vi "Flatten to String.vi"(8 "error in (no error)":errorcluster, 9 "priority":i32, 10 "Message":refnum<class "Message.lvclass">, 11 "Flattener in":refnum<class "Serializable Flattener.lvclass">) -> (0 "error out":errorcluster, 2 "Flattened String":string, 3 "Flattener out":refnum<class "Serializable Flattener.lvclass">)   [LabVIEW 2020, in "Serializer.lvlib" / "Serializable Flattener.lvclass"]
uses:
  Serializable Flattener.lvclass
  <vilib>/ActorFramework/Message/Message.lvclass
  Serializable Message/Serializable Msg.lvclass
  Cache Manager/Cache Manager.lvclass/Cache Manager.ctl
  Serializable Message/Serializable Msg.lvclass/Serializable Msg.ctl
  Serializable Message/Make Header Array.vi
  <vilib>/Utility/LVClass/Get LV Class Name.vi
  Serializable Flattener.lvclass/Serializable Flattener.ctl
  Cache Manager/Cache Manager.lvclass
panel:
  out "Elapsed time":u32
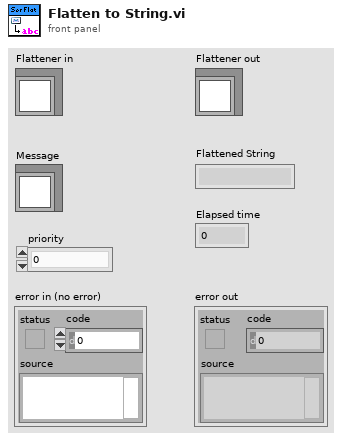
[diagram p1: front panel]
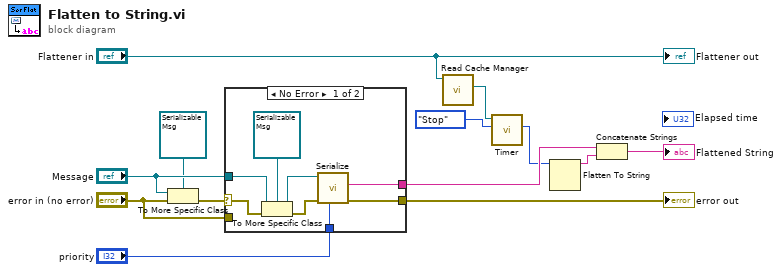
[diagram p0: block diagram]
diagram:
  n1 = To More Specific Class(target class=refnum<class "Serializable Msg.lvclass"> refnum ("Serializable Message in"), reference="Message", error in="error in (no error)") -> (error out=w9:errorcluster)  [unwired: 1 out]
  n2 = case shown="No Error" w9 {
    selector: w9 -> [w17 _]
    tunnel: [w19 w22] -> w13
    tunnel: [w18 _] -> w5
    tunnel: "Message" -> [w15 _]
    tunnel: "priority" -> [w14 _]
    tunnel: "error in (no error)" -> [_ w22]
    frame No Error {
      n3 = To More Specific Class(target class=refnum<class "Serializable Msg.lvclass"> refnum ("Serializable Message in"), reference=w15, error in=w17) -> (specific class reference=w16:refnum<class "Serializable Msg.lvclass">, error out=w21:errorcluster)
      n4 = call "Serialize.vi"("priority"=w14, "error in (no error)"=w21, "Serializable Message in"=w16) -> ("error out"=w19:errorcluster, "Serialized Message"=w18:string)  [unwired: 7 in]
    }
    frame Error {
    }
  }
  "error out" <- w13
  n5 = call-dynamic "Read Cache Manager.vi"("Message Flattener in"="Flattener in") -> ("Cache Manager DVR.lvclass"=w3:refnum<class "Cache Manager.lvclass">)  [unwired: 9 in, 1 out]
  n6 = call "Timer.vi"("Action"=enum16{"Stop", "Start", ""}."Stop", "Cache Manager DVR in"=w3) -> ("Elapsed time (ms)"=w1:u32)  [unwired: 7 in, 2 out]
  n7 = Flatten To String(anything=w1) -> (data string=w4:string)  [unwired: 3 in, 2 out]
  n8 = Concatenate Strings(w5, w4) -> (→"Flattened String":string)
  "Flattener out" <- "Flattener in"
